vi "Save SS measurement.vi"(6 "Index":i32, 7 "SS measurement":T1 {"PJVS reference voltages array of vector cluster"."PJVS reference voltages vector" format="%#_3p"; "PJVS frequencies (Hz)" format="%#_3p"; "Record lengths (multiples of periods)" format="%#_3p"; "Sampling frequencies (Hz)" format="%#_3p"; "Signal amplitudes (V)" format="%#_3p"; "Signal frequencies (Hz)" format="%#_3p"}, 8 "error in":errorcluster, 9 "Set PJVS steps":u32) -> (0 "error out":errorcluster)   [LabVIEW 2020]
doc: "Save SS measurement informations into info file."
uses:
  SS Measurement/Type definitions/SS measurement.ctl
  external libraries/TWM-1.8.7.0-client/1D EXT.vi
  external libraries/TWM-1.8.7.0-client/EXT.vi
  external libraries/TWM-1.8.7.0-client/String.vi
  external libraries/TWM-1.8.7.0-client/U64.vi
  external libraries/TWM-1.8.7.0-client/Boolean.vi
  external libraries/TWM-1.8.7.0-client/I64.vi
  external libraries/TWM-1.8.7.0-client/infolib.lvlib
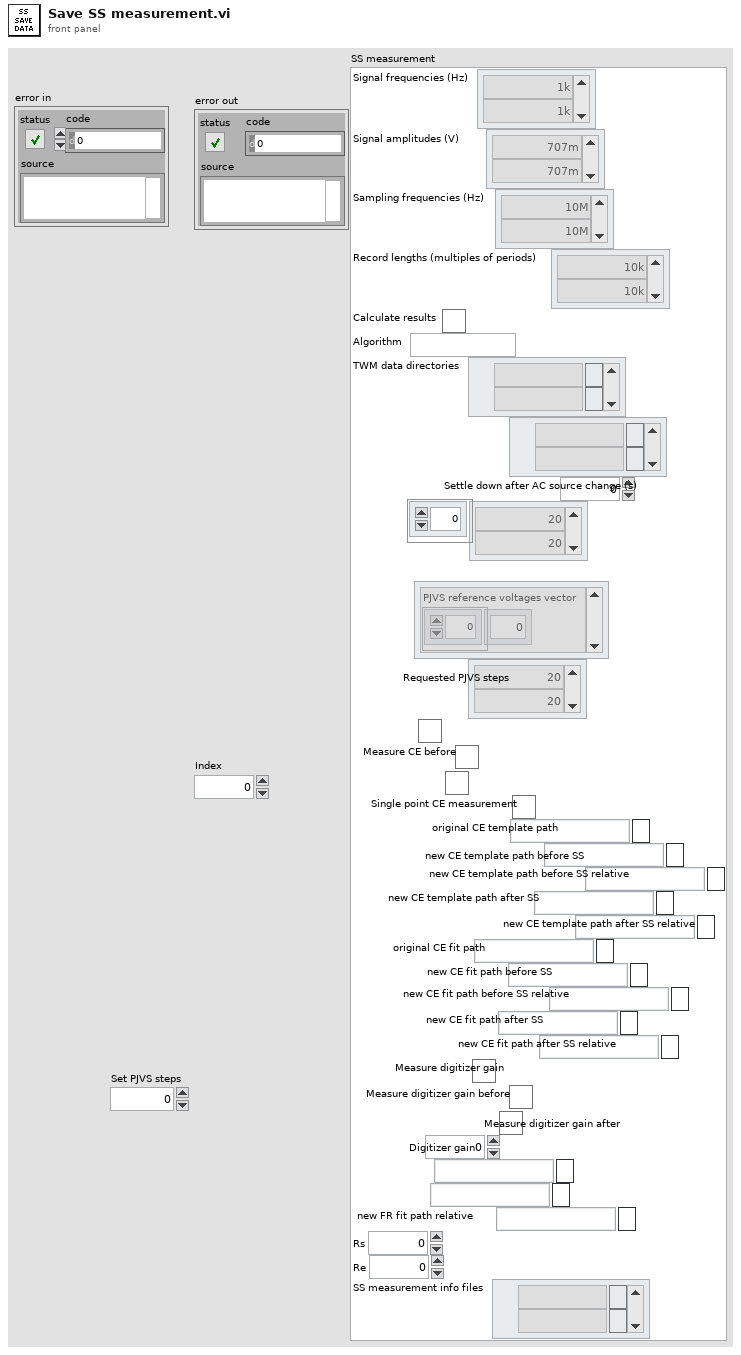
[diagram p1: front panel]
types:
  T1 = typedef "SS measurement.ctl" = cluster{"Signal frequencies (Hz)":dbl[], "Signal amplitudes (V)":dbl[], "Sampling frequencies (Hz)":dbl[], "Record lengths (multiples of periods)":dbl[], "Calculate results":bool, "Algorithm":string, "TWM data directories":path[], "TWM data directories relative":path[], "Settle down after AC source change (s)":dbl, "PJVS frequencies (Hz)":dbl[], "PJVS reference voltages array of vector cluster":cluster{"PJVS reference voltages vector":dbl[]}[], "Requested PJVS steps":u32[], "Measure CE":bool, "Measure CE before":bool, "Measure CE after":bool, "Single point CE measurement":bool, "original CE template path":path, "new CE template path before SS":path, "new CE template path before SS relative":path, "new CE template path after SS":path, "new CE template path after SS relative":path, "original CE fit path":path, "new CE fit path before SS":path, "new CE fit path before SS relative":path, "new CE fit path after SS":path, "new CE fit path after SS relative":path, "Measure digitizer gain":bool, "Measure digitizer gain before":bool, "Measure digitizer gain after":bool, "Digitizer gain":dbl, "Data folder":path, "FR fit path":path, "new FR fit path relative":path, "Rs":i32, "Re":i32, "SS measurement info files":path[]}
  T2 = cluster{"PJVS reference voltages vector":dbl[]}[]
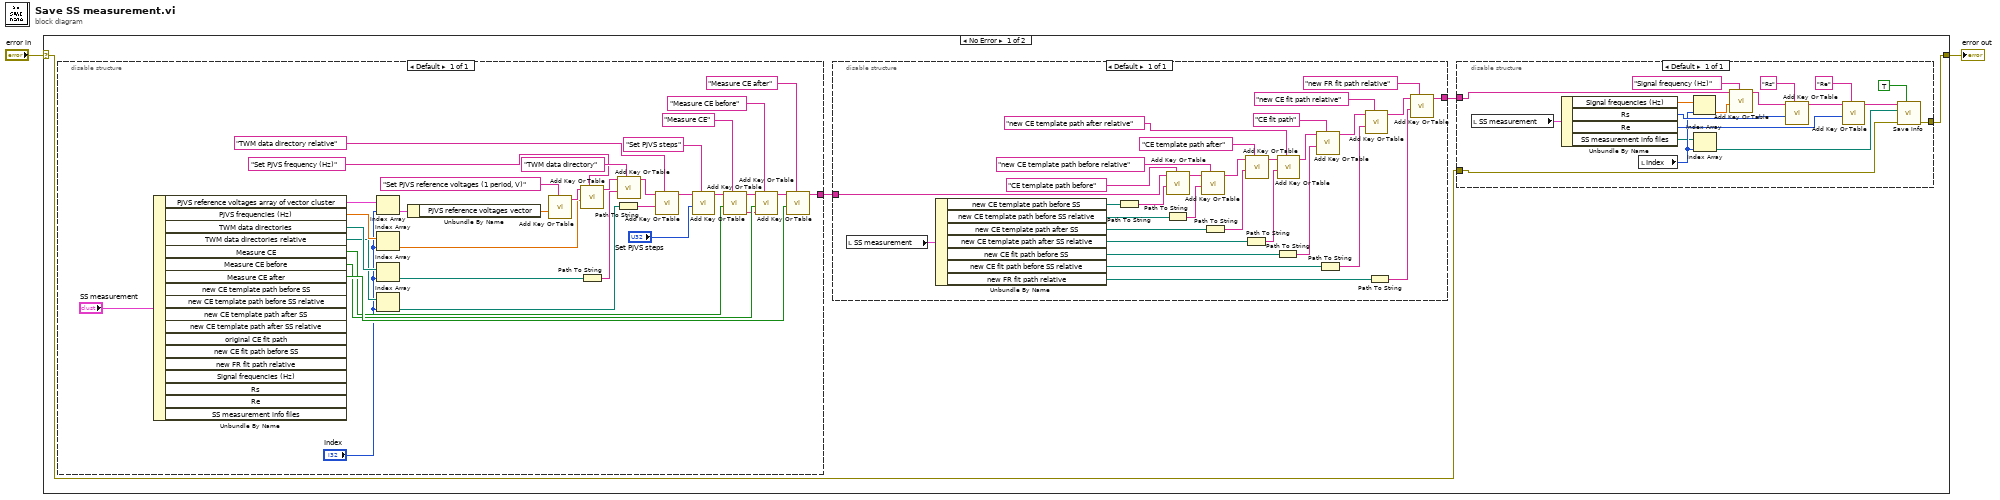
[diagram p0: block diagram]
diagram:
  n1 = case shown="No Error" "error in" {
    selector: "error in" -> [w4 w89]
    tunnel: [w5 w89] -> w2
    frame No Error {
      n2 = disable-structure shown="Default" {
        disable-tunnel: [w38] -> w6
        frame Enabled {
          n3 = Unbundle By Name("SS measurement") -> ("PJVS reference voltages array of vector cluster"=w13:T2, "PJVS frequencies (Hz)"=w15:dbl[], "TWM data directories"=w10:path[], "TWM data directories relative"=w9:path[], "Measure CE"=w20:bool, "Measure CE before"=w33:bool, "Measure CE after"=w36:bool)  [unwired: 11 out]
          n4 = Index Array(array=w13, index="Index") -> (element=w12:cluster{"PJVS reference voltages vector":dbl[]})
          n5 = Index Array(array=w15, index="Index") -> (element=w14:dbl)
          n6 = Index Array(array=w10, index="Index") -> (element=w19:path)
          n7 = Index Array(array=w9, index="Index") -> (element=w17:path)
          n8 = Unbundle By Name(w12) -> ("PJVS reference voltages vector"=w11:dbl[])
          n9 = call-poly "Add Key Or Table.vi"("key description"="Set PJVS reference voltages (1 period, V)", "numeric"=w11) -> ("info data out"=w32:string)  [unwired: 8 in, 1 out]
          n10 = call-poly "Add Key Or Table.vi"("key description"="Set PJVS frequency (Hz)", "numeric"=w14, "info data"=w32) -> ("info data out"=w31:string)  [unwired: 7 in, 1 out]
          n11 = Path To String(path=w19) -> (string=w18:string)
          n12 = Path To String(path=w17) -> (string=w16:string)
          n13 = call-poly "Add Key Or Table.vi"("key description"="TWM data directory", "string"=w18, "info data"=w31) -> ("info data out"=w23:string)  [unwired: 7 in, 1 out]
          n14 = call-poly "Add Key Or Table.vi"("key description"="TWM data directory relative", "string"=w16, "info data"=w23) -> ("info data out"=w22:string)  [unwired: 7 in, 1 out]
          n15 = call-poly "Add Key Or Table.vi"("key description"="Set PJVS steps", "numeric"="Set PJVS steps", "info data"=w22) -> ("info data out"=w25:string)  [unwired: 7 in, 1 out]
          n16 = call-poly "Add Key Or Table.vi"("key description"="Measure CE", "boolean"=w20, "info data"=w25) -> ("sections out"=w27:string[], "info data out"=w26:string)  [unwired: 7 in]
          n17 = call-poly "Add Key Or Table.vi"("key description"="Measure CE before", "sections"=w27, "boolean"=w33, "info data"=w26) -> ("info data out"=w37:string)  [unwired: 6 in, 1 out]
          n18 = call-poly "Add Key Or Table.vi"("key description"="Measure CE after", "boolean"=w36, "info data"=w37) -> ("info data out"=w38:string)  [unwired: 7 in, 1 out]
        }
      }
      n19 = disable-structure shown="Default" {
        disable-tunnel: w6 -> [w67]
        disable-tunnel: [w49] -> w3
        frame Enabled {
          n20 = local read "SS measurement"() -> (w41:T1)
          n21 = Unbundle By Name(w41) -> ("new CE template path before SS"=w43:path, "new CE template path before SS relative"=w48:path, "new CE template path after SS"=w42:path, "new CE template path after SS relative"=w47:path, "new CE fit path before SS"=w46:path, "new CE fit path before SS relative"=w45:path, "new FR fit path relative"=w44:path)
          n22 = Path To String(path=w43) -> (string=w68:string)
          n23 = Path To String(path=w48) -> (string=w69:string)
          n24 = call-poly "Add Key Or Table.vi"("key description"="CE template path before", "string"=w68, "info data"=w67) -> ("info data out"=w70:string)  [unwired: 7 in, 1 out]
          n25 = call-poly "Add Key Or Table.vi"("key description"="new CE template path before relative", "string"=w69, "info data"=w70) -> ("info data out"=w66:string)  [unwired: 7 in, 1 out]
          n26 = Path To String(path=w42) -> (string=w65:string)
          n27 = Path To String(path=w47) -> (string=w61:string)
          n28 = call-poly "Add Key Or Table.vi"("key description"="CE template path after", "string"=w65, "info data"=w66) -> ("info data out"=w64:string)  [unwired: 7 in, 1 out]
          n29 = Path To String(path=w46) -> (string=w60:string)
          n30 = call-poly "Add Key Or Table.vi"("key description"="new CE template path after relative", "string"=w61, "info data"=w64) -> ("info data out"=w63:string)  [unwired: 7 in, 1 out]
          n31 = call-poly "Add Key Or Table.vi"("key description"="CE fit path", "string"=w60, "info data"=w63) -> ("info data out"=w62:string)  [unwired: 7 in, 1 out]
          n32 = Path To String(path=w45) -> (string=w59:string)
          n33 = call-poly "Add Key Or Table.vi"("key description"="new CE fit path relative", "string"=w59, "info data"=w62) -> ("info data out"=w50:string)  [unwired: 7 in, 1 out]
          n34 = Path To String(path=w44) -> (string=w51:string)
          n35 = call-poly "Add Key Or Table.vi"("key description"="new FR fit path relative", "string"=w51, "info data"=w50) -> ("info data out"=w49:string)  [unwired: 7 in, 1 out]
        }
      }
      n36 = disable-structure shown="Default" {
        disable-tunnel: [w87] -> w5
        disable-tunnel: w4 -> [w86]
        disable-tunnel: w3 -> [w84]
        frame Enabled {
          n37 = local read "SS measurement"() -> (w72:T1)
          n38 = Unbundle By Name(w72) -> ("Signal frequencies (Hz)"=w76:dbl[], "Rs"=w75:i32, "Re"=w74:i32, "SS measurement info files"=w71:path[])
          n39 = local read "Index"() -> (w73:i32)
          n40 = Index Array(array=w76, index=w73) -> (element=w77:dbl)
          n41 = Index Array(array=w71, index=w73) -> (element=w78:path)
          n42 = call-poly "Add Key Or Table.vi"("key description"="Signal frequency (Hz)", "numeric"=w77, "info data"=w84) -> ("info data out"=w80:string)  [unwired: 7 in, 1 out]
          n43 = call-poly "Add Key Or Table.vi"("key description"="Rs", "numeric"=w75, "info data"=w80) -> ("info data out"=w81:string)  [unwired: 7 in, 1 out]
          n44 = call-poly "Add Key Or Table.vi"("key description"="Re", "numeric"=w74, "info data"=w81) -> ("info data out"=w79:string)  [unwired: 7 in, 1 out]
          n45 = call "Save Info.vi"("Overwrite? (T)"=TRUE, "error in"=w86, "filename"=w78, "info data"=w79) -> ("error out"=w87:errorcluster)  [unwired: 7 in]
        }
      }
    }
    frame Error {
    }
  }
  "error out" <- w2
